vi "Evaluate Part 1.vi"() -> ()   [LabVIEW 2020]
uses:
  Map/Map.lvclass
panel:
  out "Locations":i32[](array[numeric])=[82, 43, 86, 35]
  in  "Input":string="seeds: 79 14 55 13\n\nseed-to-soil map:\n50 98 2\n52 50 48\n\nsoil-to-fertilizer map:\n0 15 37\n37 52 2\n39 0 15\n\nfertilizer-to-water map:\n49 53 8\n0 11 42\n42 0 7\n57 7 4\n\nwater-to-light map:\n88 18 7\n18 25 70\n\nlight-to-temperature map:\n45 77 23\n81 45 19\n68 64 13\n\ntemperature-to-humidity map:\n0 69 1\n1 0 69\n\nhumidity-to-location map:\n60 56 37\n56 93 4"
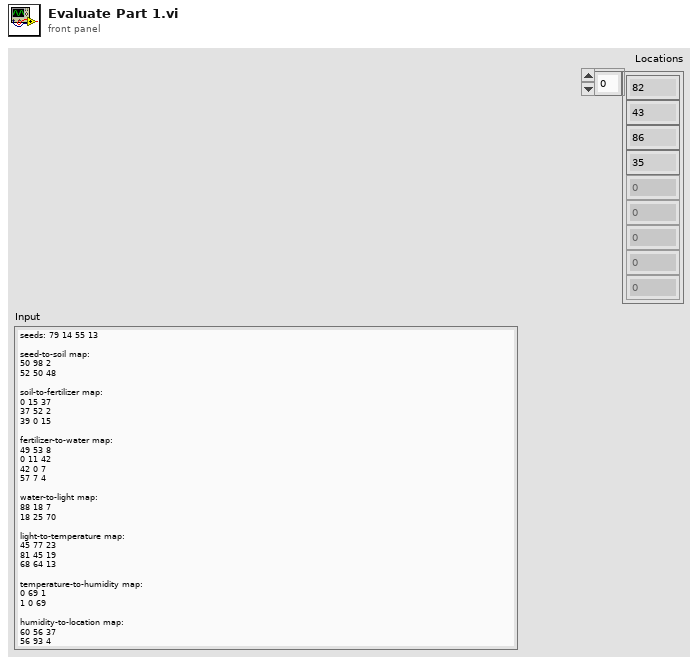
[diagram p1: front panel]
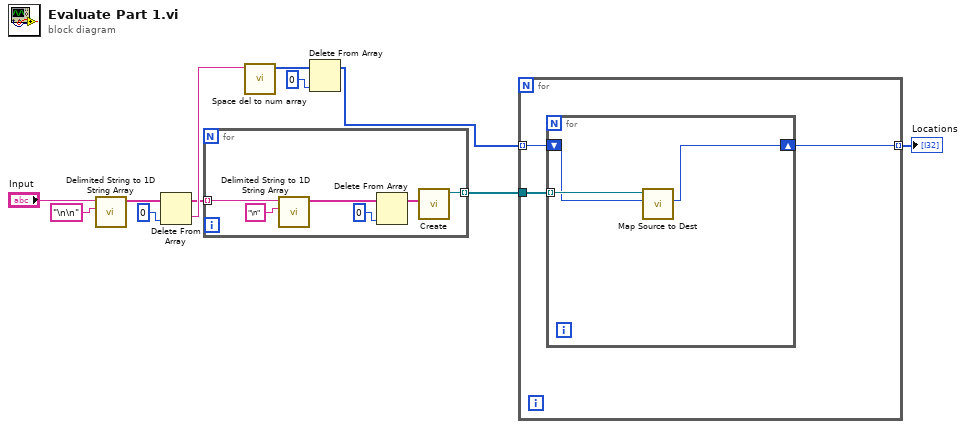
[diagram p0: block diagram]
diagram:
  n1 = call <vilib>:"Delimited String to 1D String Array.vi"("delimiter"="\n\n" ("String"), "delimited string"="Input") -> ("string array"=w5:string[])  [unwired: 9 in]
  n2 = Delete From Array(array=w5, index=0) -> (deleted portion=w8:string, array with subset deleted=w4:string[])  [unwired: 1 in]
  n3 = for {
    tunnel: w4 -> [w15] mode=indexing
    tunnel: [w12] -> w3 mode=indexing
    n4 = call <vilib>:"Delimited String to 1D String Array.vi"("delimiter"="\n" ("String"), "delimited string"=w15) -> ("string array"=w14:string[])  [unwired: 9 in]
    n5 = Delete From Array(array=w14, index=0) -> (array with subset deleted=w13:string[])  [unwired: 1 in, 1 out]
    n6 = call "Create.vi"("Input"=w13) -> ("Map"=w12:refnum<class "Map.lvclass">)  [unwired: 9 in, 1 out]
  }
  n7 = call "Space del to num array.vi"("Input in"=w8) -> ("Input out"=w7:i32[])  [unwired: 10 in]
  n8 = Delete From Array(array=w7, index=0) -> (array with subset deleted=w2:i32[])  [unwired: 1 in, 1 out]
  n9 = for {
    tunnel: w3 -> [w20]
    tunnel: w2 -> [w19] mode=indexing
    tunnel: [w18] -> w1 mode=indexing
    n10 = for {
      tunnel: w20 -> [w23] mode=indexing
      shift-right: [w21] -> w18
      shift-left: w19 -> [w22]
      n11 = call "Map Source to Dest.vi"("Source"=w22, "Map in"=w23) -> ("Destination"=w21:i32)  [unwired: 7 in, 2 out]
    }
  }
  "Locations" <- w1
